vi "add_QuaternionStamped_roslv.vi"(5 "Quaternion":cluster{"x":dbl, "y":dbl, "z":dbl, "w":dbl}, 6 "Stamp":cluster{"frame_id":string, "reset seq?":bool}, 7 "msg in":string) -> (3 "msg out":string)   [LabVIEW 2014]
doc: "Flattens a quaternion stamped into a message"
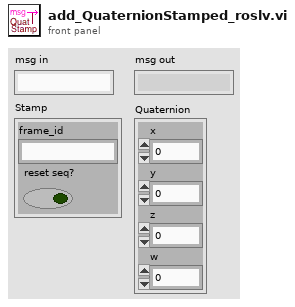
[diagram p1: front panel]
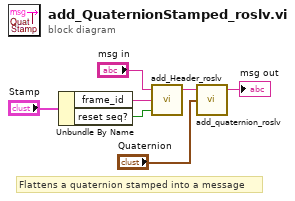
[diagram p0: block diagram]
diagram:
  # "Flattens a quaternion stamped into a message"
  n1 = Unbundle By Name("Stamp") -> ("frame_id"=w3:string, "reset seq?"=w2:bool)
  n2 = call "add_Header_roslv.vi"("reset seq?"=w2, "frame_id"=w3, "msg in"="msg in") -> ("msg out"=w5:string)  [unwired: 2 in]
  n3 = call "add_quaternion_roslv.vi"("Quaternion"="Quaternion", "msg in"=w5) -> ("msg out"=→"msg out":string)  [unwired: 3 in]
